vi "RT Main_V1.vi"() -> ()   [LabVIEW 2017]
doc: "This template is for the Queued Message Handler design pattern.\n\nThe Event Handling Loop generates messages based on user interface actions.\n\nThe Message Handling Loop processes messages generated by the Event Handling Loop, or by other messages. The messages are string values, so new messages can be added easily to the Message Cases case structure in the Message Handling Loop. Each message cluster can also provide an optional value for Message Data, which is a variant that can be converted to whatever message-specific data is required."
uses:
  UI Error Handlers/support/Message Queue/Message Queue.lvlib
  Globals/Global - All RT Loop Stop.vi
  <vilib>/rvi/interface/nirviReadWriteControl/nirviReadWriteControl.xnode
  <vilib>/rvi/errors/niLvFpgaAdjustHostInterfaceError.vi
  controls/FPGA State.ctl
  Globals/Global - Configuration Options.vi
  Globals/Global - RT Stream Connections.vi
  NiFpgaLv.dll
  <vilib>/rvi/interface/Simulation/niFpgaSimulationCallBeginRW.vi
  <vilib>/nisyscfg/nisyscfg.lvlib
  controls/Chatter data.ctl
panel:
  in  "Boolean 2":bool
  out "Boolean":bool=TRUE
  out "G1 status":cluster{"G1 ":bool}
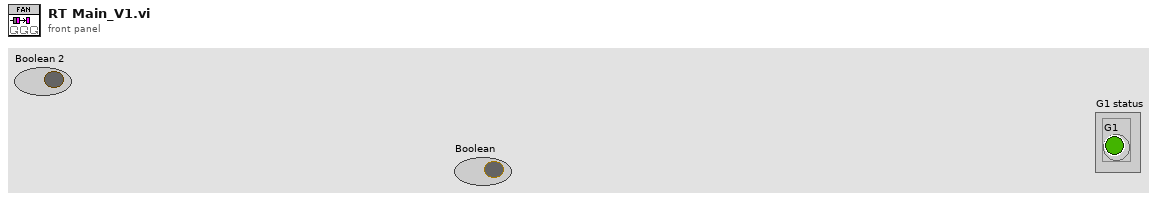
[diagram p1: front panel]
types:
  T1 = typedef "Acceleration RT FIFO Reference.ctl" = refnum<k33>
  T2 = typedef "FPGA State.ctl" = enum16{"Safe State", "Control (PID)"}
  T3 = typedef "Chatter data.ctl" = cluster{"Tool data":cluster{"Number of teeth":sgl}, "Cutting data":cluster{"rpm":sgl}, "Limits":cluster{"Magnitude threshold":sgl, "Tolerance":sgl}, "G1 status":cluster{"G1 ":bool}}
  T4 = cluster{"FPGA State":T2, "Max Acceleration Threshold":sgl, "Chatter Data":T3}
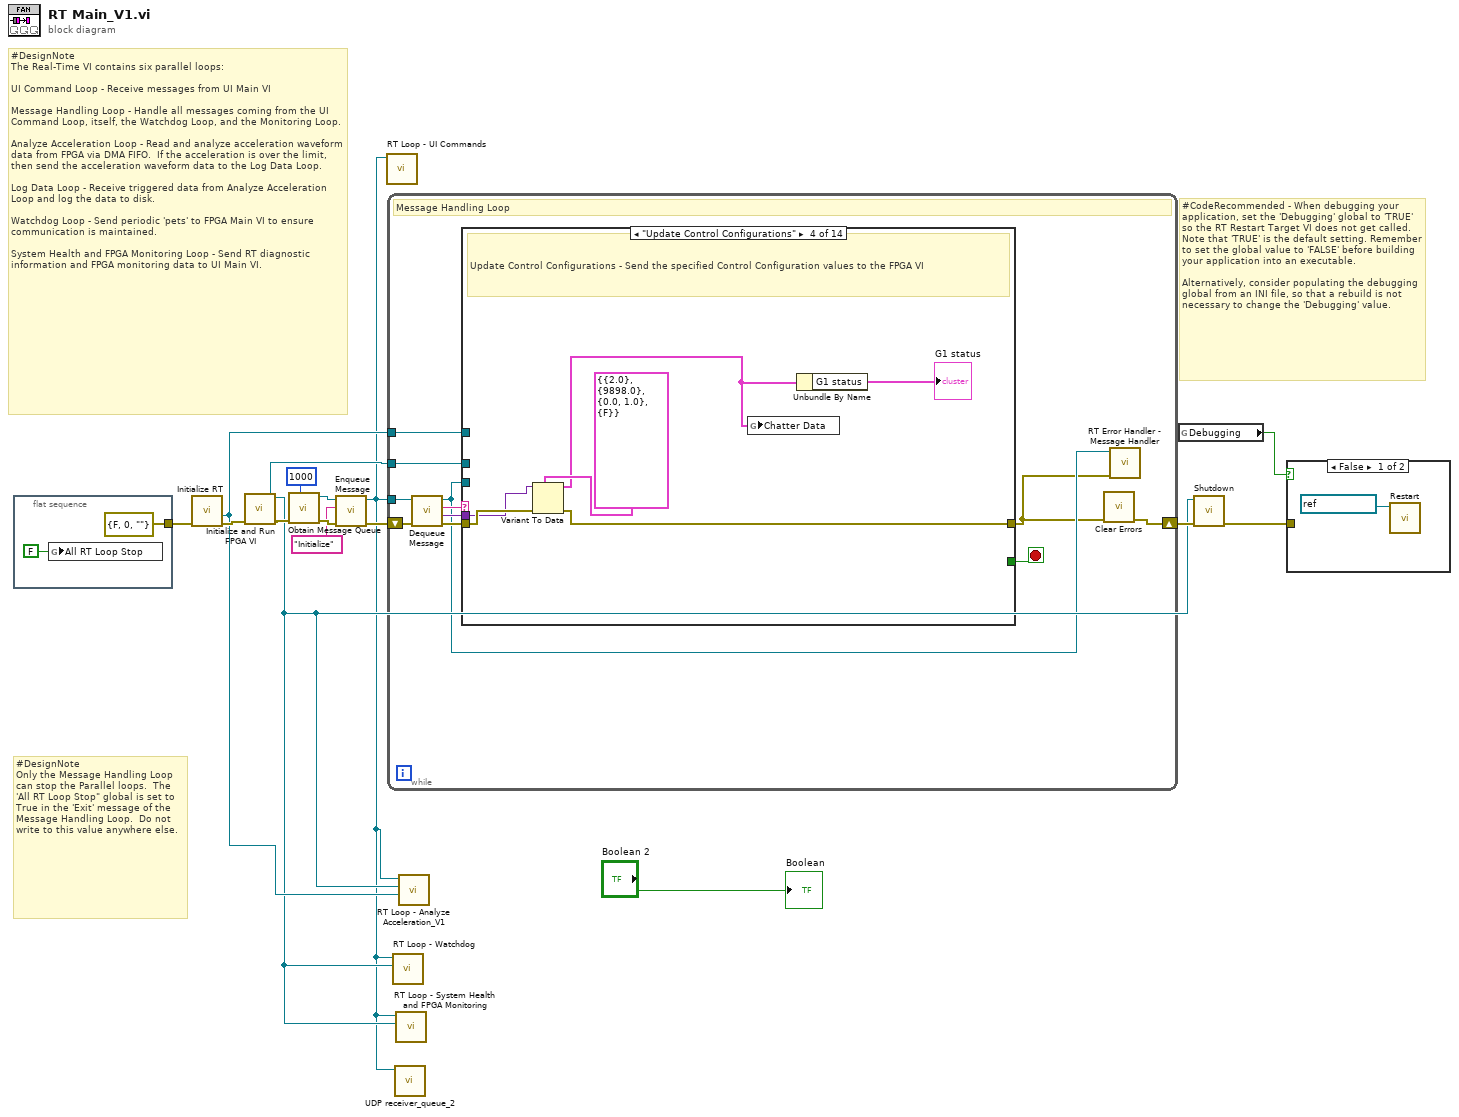
[diagram p0: block diagram]
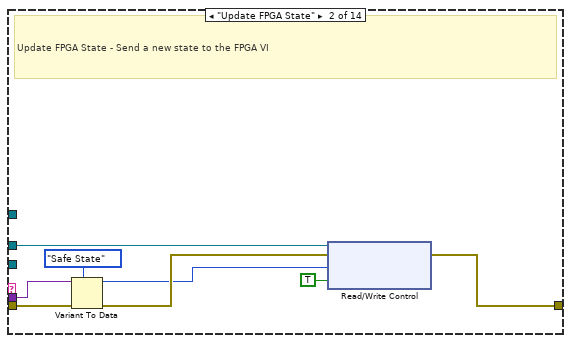
[diagram p4: hidden frame]
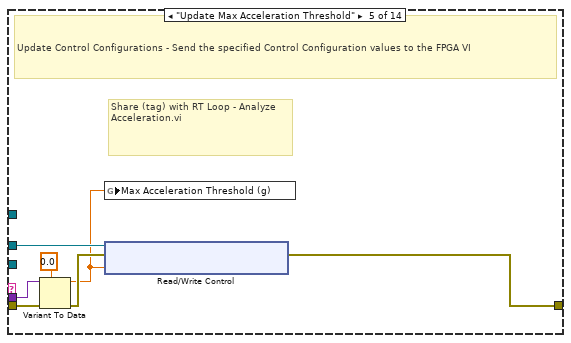
[diagram p6: hidden frame]
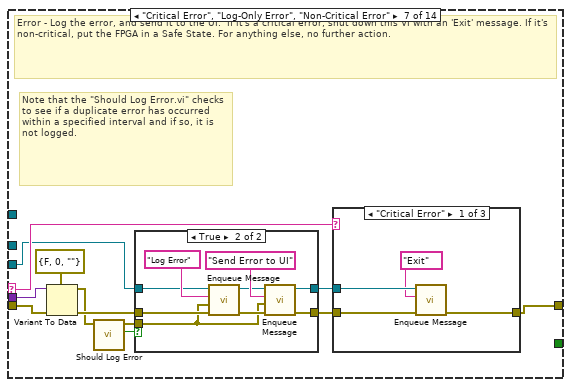
[diagram p8: hidden frame]
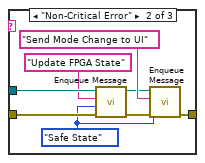
[diagram p10: hidden frame]
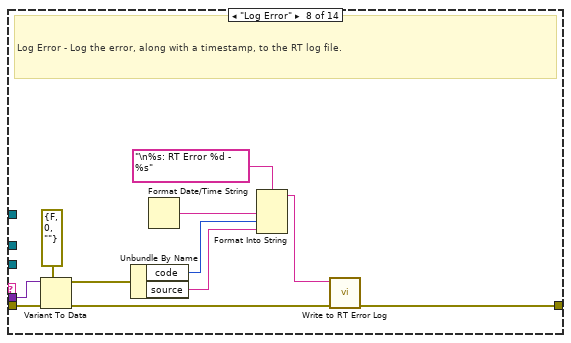
[diagram p12: hidden frame]
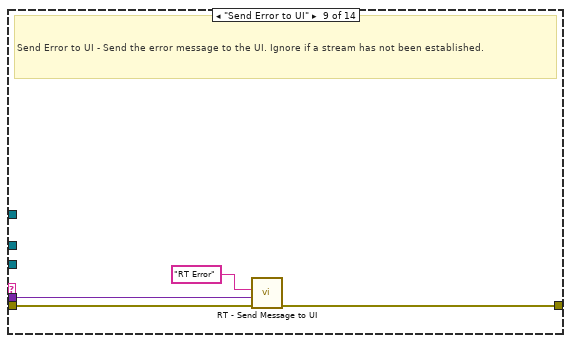
[diagram p13: hidden frame]
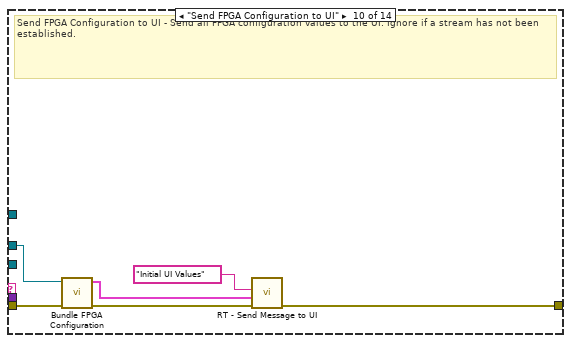
[diagram p14: hidden frame]
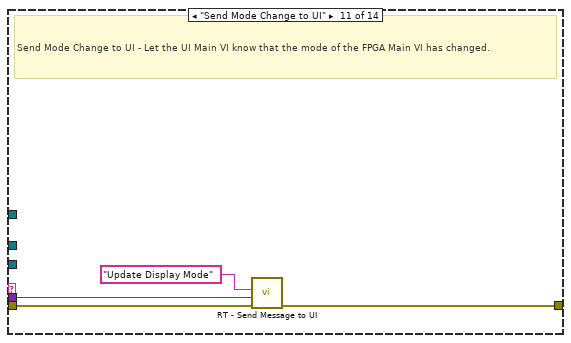
[diagram p15: hidden frame]
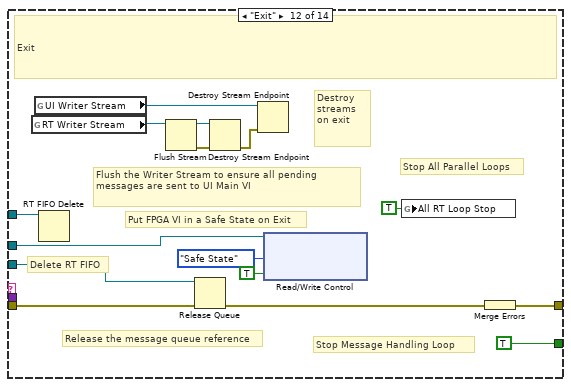
[diagram p16: hidden frame]
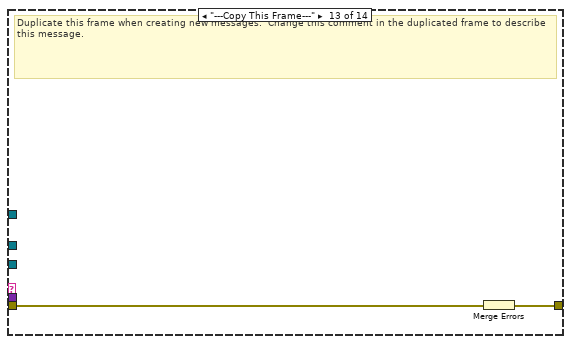
[diagram p17: hidden frame]
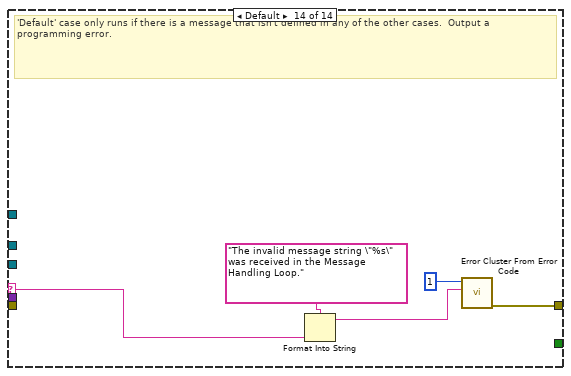
[diagram p18: hidden frame]
diagram:
  # "#CodeRecommended - When debugging your application, set the 'Debugging' global to 'TRUE' so the RT Restart Target VI does not get called.  Note that 'TRUE' is the default setting. Remember to set the global value to 'FALSE' before building your application into an executable.\n\nAlternatively, consider populating the debugging global from an INI file, so that a rebuild is not necessary to change the 'Debugging' value."
  # "#DesignNote\nThe Real-Time VI contains six parallel loops:\n\nUI Command Loop - Receive messages from UI Main VI\n\nMessage Handling Loop - Handle all messages coming from the UI Command Loop, itself, the Watchdog Loop, and the Monitoring Loop.\n\nAnalyze Acceleration Loop - Read and analyze acceleration waveform data from FPGA via DMA FIFO.  If the acceleration is over the limit, then send the acceleration waveform data to the Log Data Loop.\n\nLog Data Loop - Receive triggered data from Analyze Acceleration Loop and log the data to disk.\n\nWatchdog Loop - Send periodic 'pets' to FPGA Main VI to ensure communication is maintained.\n\nSystem Health and FPGA Monitoring Loop - Send RT diagnostic information and FPGA monitoring data to UI Main VI."
  # "#DesignNote\nOnly the Message Handling Loop can stop the Parallel loops.  The 'All RT Loop Stop\" global is set to True in the 'Exit' message of the Message Handling Loop.  Do not write to this value anywhere else."
  n1 = flat-sequence {
    tunnel: [errorcluster {"status"=FALSE, "code"=0, "source"=""} ("error constant")] -> w7
    frame #0 {
      n2 = global write "Global - All RT Loop Stop.vi" "All RT Loop Stop"(FALSE) -> ()
    }
  }
  n3 = call "Initialize RT.vi"("error in"=w7) -> ("error out"=w8:errorcluster, "Acceleration RT FIFO"=w4:T1)  [unwired: 8 in, 1 out]
  n4 = call "Initialize and Run FPGA VI.vi"("error in (no error)"=w8) -> ("error out"=w11:errorcluster, "FPGA VI Reference Out 2"=w3:refnum<k20>)  [unwired: 9 in]
  n5 = call "Obtain Message Queue.vi"("max queue size (-1, unlimited)"=1000, "error in (no error)"=w11) -> ("error out"=w15:errorcluster, "Message Queue"=w14:refnum<queue>)  [unwired: 8 in]
  n6 = call "Enqueue Message.vi"("error in (no error)"=w15, "Message"="Initialize", "Message Queue"=w14) -> ("error out"=w12:errorcluster, "dup Message Queue"=w2:refnum<queue>)  [unwired: 7 in]
  n7 = call "RT Loop - UI Commands.vi"("Message Queue"=w2) -> ()  [unwired: 11 in]
  n8 = while {
    tunnel: w2 -> [w23]
    shift-right: [w20] -> w6
    shift-left: w12 -> [w27]
    tunnel: w3 -> [w22]
    tunnel: w4 -> [w18]
    stop <- w28 stop-if-true
    # "Message Handling Loop"
    n9 = call "Dequeue Message.vi"("error in (no error)"=w27, "Message Queue"=w23) -> ("error out"=w26:errorcluster, "Message Data"=w24:variant, "Message"=w25:string, "dup Message Queue"=w21:refnum<queue>)  [unwired: 6 in]
    n10 = case "Message Cases" shown="\"Update Control Configurations\"" w25 {
      selector: w25 -> [_ _ _ _ _ _ w62 _ _ _ _ _ _ w134]
      tunnel: w21 -> [_ _ _ _ _ _ w56 _ _ _ _ w128 _ _]
      tunnel: w26 -> [w29 w37 w38 w44 w51 w52 w60 w99 w103 w109 w113 w124 w130 _]
      tunnel: [w29 w34 w38 w43 w45 w52 w61 w90 w100 w106 w112 w125 w129 w132] -> w19
      tunnel: [_ _ _ _ _ _ _ _ _ _ _ TRUE _ _] -> w28
      tunnel: w24 -> [_ w36 _ w42 w50 _ w59 w98 w102 _ w111 _ _ _]
      tunnel: w22 -> [_ w32 _ _ w48 _ _ _ _ w105 _ w120 _ _]
      tunnel: w18 -> [_ _ _ _ _ _ _ _ _ _ _ w114 _ _]
      frame "Initialize" {
        # "Initialize - Currently a no-op for the RT Main VI"
      }
      frame "Update FPGA State" {
        # "Update FPGA State - Send a new state to the FPGA VI"
        n11 = Variant To Data(error in=w37, type=FPGA_State."Safe State" ("FPGA State"), Variant=w36) -> (data=w31:T2, error out=w33:errorcluster)
        n12 = xnode "Read/Write Control"("FPGA VI Reference In"=w32, "error in"=w33, "New FPGA State"=w31, "Change State"=TRUE) -> ("error out"=w34:errorcluster)  [unwired: 1 out]
      }
      frame "Update Setpoints" {
        # "Update Setpoints - Send the specified setpoint values to the FPGA VI"
      }
      frame "Update Control Configurations" {
        # "Update Control Configurations - Send the specified Control Configuration values to the FPGA VI"
        n13 = Variant To Data(error in=w44, type=T3 {"Tool data"={"Number of teeth"=2.0}, "Cutting data"={"rpm"=9898.0}, "Limits"={"Magnitude threshold"=0.0, "Tolerance"=1.0}, "G1 status"={"G1 "=FALSE}} ("Chatter Data"), Variant=w42) -> (data=w40:T3, error out=w43:errorcluster)
        n14 = global write "Global - Configuration Options.vi" "Chatter Data"(w40) -> ()
        n15 = Unbundle By Name(w40) -> ("G1 status"=→"G1 status":cluster{"G1 ":bool})
      }
      frame "Update Max Acceleration Threshold" {
        # "Share (tag) with RT Loop - Analyze Acceleration.vi"
        # "Update Control Configurations - Send the specified Control Configuration values to the FPGA VI"
        n16 = Variant To Data(error in=w51, type=sgl 0.0 ("SGL"), Variant=w50) -> (data=w46:sgl, error out=w49:errorcluster)
        n17 = global write "Global - Configuration Options.vi" "Max Acceleration Threshold (g)"(w46) -> ()
        n18 = xnode "Read/Write Control"("FPGA VI Reference In"=w48, "error in"=w49, "Max Acceleration Threshold (g)"=w46) -> ("error out"=w45:errorcluster)  [unwired: 1 out]
      }
      frame "Update Max Fan Speed Threshold" {
        # "Update Control Configurations - Send the specified Control Configuration values to the FPGA VI"
      }
      frame "Critical Error", "Log-Only Error", "Non-Critical Error" {
        # "Note that the \"Should Log Error.vi\" checks to see if a duplicate error has occurred within a specified interval and if so, it is not logged."
        # "Error - Log the error, and send it to the UI.  If it's a critical error, shut down this VI with an 'Exit' message. If it's non-critical, put the FPGA in a Safe State. For anything else, no further action."
        n19 = Variant To Data(error in=w60, type=errorcluster {"status"=FALSE, "code"=0, "source"=""} ("error out"), Variant=w59) -> (data=w54:errorcluster, error out=w57:errorcluster)
        n20 = call "Should Log Error.vi"("error to report"=w54) -> ("Should Log Error?"=w55:bool, "dup error to report"=w53:errorcluster)  [unwired: 9 in]
        n21 = case shown="True" w55 {
          tunnel: [w66 w73] -> w64
          tunnel: [w65 w72] -> w63
          tunnel: w56 -> [w65 w71]
          tunnel: w57 -> [w66 w68]
          tunnel: w53 -> [_ w67]
          frame False {
          }
          frame True {
            n22 = call "Enqueue Message.vi"("error in (no error)"=w68, "Message Data"=w67, "Message"="Log Error", "Message Queue"=w71) -> ("error out"=w69:errorcluster, "dup Message Queue"=w70:refnum<queue>)  [unwired: 6 in]
            n23 = call "Enqueue Message.vi"("error in (no error)"=w69, "Message Data"=w67, "Message"="Send Error to UI", "Message Queue"=w70) -> ("error out"=w73:errorcluster, "dup Message Queue"=w72:refnum<queue>)  [unwired: 6 in]
          }
        }
        n24 = case shown="\"Critical Error\"" w62 {
          tunnel: w64 -> [w79 w87 w88]
          tunnel: w63 -> [w77 w86 _]
          tunnel: [w78 w83 w88] -> w61
          frame "Critical Error" {
            n25 = call "Enqueue Message.vi"("error in (no error)"=w79, "Message"="Exit", "Message Queue"=w77) -> ("error out"=w78:errorcluster)  [unwired: 7 in, 1 out]
          }
          frame "Non-Critical Error" {
            w80 = FPGA_State."Safe State" ("FPGA State")
            n26 = call "Enqueue Message.vi"("error in (no error)"=w87, "Message Data"=w80, "Message"="Update FPGA State", "Message Queue"=w86) -> ("error out"=w84:errorcluster, "dup Message Queue"=w81:refnum<queue>)  [unwired: 6 in]
            n27 = call "Enqueue Message.vi"("error in (no error)"=w84, "Message Data"=w80, "Message"="Send Mode Change to UI", "Message Queue"=w81) -> ("error out"=w83:errorcluster)  [unwired: 6 in, 1 out]
          }
          frame Default {
          }
        }
      }
      frame "Log Error" {
        # "Log Error - Log the error, along with a timestamp, to the RT log file."
        n28 = Variant To Data(error in=w99, type=errorcluster {"status"=FALSE, "code"=0, "source"=""} ("error constant"), Variant=w98) -> (data=w93:errorcluster, error out=w96:errorcluster)
        n29 = Unbundle By Name(w93) -> ("code"=w92:i32, "source"=w91:string)
        n30 = Format Date/Time String() -> (date/time string=w94:string)  [unwired: 3 in]
        n31 = Format Into String(format string="\n%s: RT Error %d - %s", w94, w92, w91) -> (resulting string=w89:string)  [unwired: 2 in, 1 out]
        n32 = call "Write to RT Error Log.vi"("error in (no error)"=w96, "Log Entry"=w89) -> ("error out"=w90:errorcluster)  [unwired: 9 in]
      }
      frame "Send Error to UI" {
        # "Send Error to UI - Send the error message to the UI. Ignore if a stream has not been established."
        n33 = call "RT - Send Message to UI.vi"("error in (no error)"=w103, "Message Data"=w102, "Message"="RT Error") -> ("error out"=w100:errorcluster)  [unwired: 8 in]
      }
      frame "Send FPGA Configuration to UI" {
        # "Send FPGA Configuration to UI - Send all FPGA configuration values to the UI. Ignore if a stream has not been established."
        n34 = call "Bundle FPGA Configuration.vi"("error in (no error)"=w109, "FPGA VI Reference Out 2"=w105) -> ("error out"=w108:errorcluster, "Cluster"=w104:T4)  [unwired: 8 in]
        n35 = call "RT - Send Message to UI.vi"("error in (no error)"=w108, "Message Data"=w104, "Message"="Initial UI Values") -> ("error out"=w106:errorcluster)  [unwired: 8 in]
      }
      frame "Send Mode Change to UI" {
        # "Send Mode Change to UI - Let the UI Main VI know that the mode of the FPGA Main VI has changed."
        n36 = call "RT - Send Message to UI.vi"("error in (no error)"=w113, "Message Data"=w111, "Message"="Update Display Mode") -> ("error out"=w112:errorcluster)  [unwired: 8 in]
      }
      frame "Exit" {
        # "Delete RT FIFO"
        # "Flush the Writer Stream to ensure all pending messages are sent to UI Main VI"
        # "Destroy streams on exit"
        # "Put FPGA VI in a Safe State on Exit"
        # "Stop Message Handling Loop"
        # "Stop All Parallel Loops"
        # "Release the message queue reference"
        # "Exit"
        n37 = global read "Global - RT Stream Connections.vi" "RT Writer Stream"() -> (w117:refnum<k21>)
        n38 = global read "Global - RT Stream Connections.vi" "UI Writer Stream"() -> (w119:refnum<k21>)
        n39 = RT FIFO Delete(0:w114) -> ()  [unwired: 2 in, 1 out]
        n40 = Flush Stream(11:w117) -> (0:w115:errorcluster, 3:w116:refnum<k21>)  [unwired: 3 in, 1 out]
        n41 = Release Queue(queue=w128, error in (no error)=w124) -> (error out=w126:errorcluster)  [unwired: 1 in, 2 out]
        n42 = Destroy Stream Endpoint(8:w115, 11:w116) -> (0:w118:errorcluster)
        n43 = Destroy Stream Endpoint(8:w118, 11:w119) -> ()  [unwired: 1 out]
        n44 = xnode "Read/Write Control"("FPGA VI Reference In"=w120, "New FPGA State"=FPGA_State."Safe State" ("New State"), "Change State"=TRUE) -> ()  [unwired: 1 in, 2 out]
        n45 = global write "Global - All RT Loop Stop.vi" "All RT Loop Stop"(TRUE ("Stop Monitoring Loops")) -> ()
        n46 = Merge Errors(w126) -> (w125:errorcluster)
      }
      frame "---Copy This Frame---" {
        # "Duplicate this frame when creating new messages.  Change this comment in the duplicated frame to describe this message."
        n47 = Merge Errors(w130) -> (w129:errorcluster)
      }
      frame Default {
        # "'Default' case only runs if there is a message that isn't defined in any of the other cases.  Output a programming error."
        n48 = Format Into String(format string="The invalid message string \"%s\" was received in the Message Handling Loop." ("Unknown Message Error Text"), w134) -> (resulting string=w131:string)  [unwired: 2 in, 1 out]
        n49 = call <vilib>:"Error Cluster From Error Code.vi"("error message (\"\")"=w131, "error code (0)"=1) -> ("error out"=w132:errorcluster)  [unwired: 7 in]
      }
    }
    n50 = call <vilib>:"Clear Errors.vi"("error in (no error)"=w19) -> ("error out"=w20:errorcluster)  [unwired: 5 in, 1 out]
    n51 = call "RT Error Handler - Message Handler.vi"("error in (no error)"=w19, "Message Queue"=w21) -> ()  [unwired: 9 in, 1 out]
  }
  n52 = call "RT Loop - Watchdog.vi"(10:w3, "Message Queue"=w2) -> ()  [unwired: 10 in]
  n53 = call "UDP receiver_queue_2.vi"("dup Message Queue"=w2) -> ()  [unwired: 11 in]
  n54 = call "RT Loop - System Health and FPGA Monitoring.vi"("FPGA VI Reference Out 2"=w3, "Message Queue"=w2) -> ()  [unwired: 10 in]
  n55 = call "RT Loop - Analyze Acceleration_V1.vi"("Acceleration RT FIFO In"=w4, "FPGA VI Reference Out 2"=w3, "Message Queue"=w2) -> ()  [unwired: 8 in, 1 out]
  n56 = global read "Global - Configuration Options.vi" "Debugging"() -> (w10:bool)
  n57 = call "Shutdown.vi"("error in"=w6, "FPGA VI Reference in"=w3) -> ("error out"=w5:errorcluster)  [unwired: 9 in]
  n58 = case shown="False" w10 {
    tunnel: w5 -> [_ _]
    frame False {
      n59 = call <vilib>:"Restart.vi"("Session in"=refnum<k21> "localhost" ("session in")) -> ()  [unwired: 8 in, 3 out]
    }
    frame True {
    }
  }
  "Boolean" <- "Boolean 2"
